vi "Read Persistent Layers.vi"(11 "Attributes in":refnum<class "Attributes.lvclass">) -> (2 "Persistent Layers":refnum<class "Actor.lvclass">[](array[class]))   [LabVIEW 2025, in "jettl.lvlib" / "Attributes.lvclass"]
uses:
  Attributes.lvclass
  Actor/Actor.lvclass
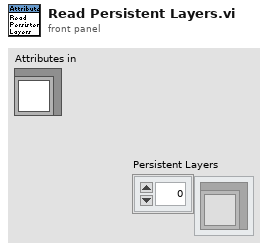
[diagram p1: front panel]
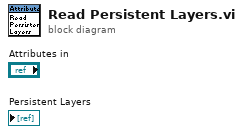
[diagram p0: block diagram]
diagram:
